vi "LidarEncoder (SubVI).vi"(10 "Direction":dbl[](array[numeric]), 11 "Magnitude":dbl[](array[numeric])) -> (2 "Encoded":T1)   [LabVIEW 2014]
types:
  T1 = cluster{"Magnitude":u16[], "Direction":fxp<+/-,16,8>[]}
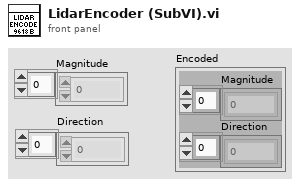
[diagram p1: front panel]
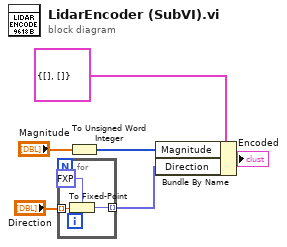
[diagram p0: block diagram]
diagram:
  n1 = for {
    tunnel: "Direction" -> [w9] mode=indexing
    tunnel: [w7] -> w1 mode=indexing
    n2 = To Fixed-Point(fixed-point type=fxp<+/-,16,8> 0.0, number=w9) -> (fixed-point=w7:fxp<+/-,16,8>)
  }
  n3 = To Unsigned Word Integer(number="Magnitude") -> (unsigned 16bit integer=w3:u16[])
  n4 = Bundle By Name(cluster=T1 {"Magnitude"=[], "Direction"=[]} ("notification in"), "Magnitude"=w3, "Direction"=w1) -> (→"Encoded":T1)
